vi "NicmosReverseScan.vi"(3 "Scan":T1, 7 "Reverse":bool, 9 "error out":errorcluster caption="error in (no error)") -> (0 "Reversed Scan":T1, 6 "error in (no error)":errorcluster caption="error out")   [LabVIEW 2009]
uses:
  Controls/NICMOS.DATA.ctl
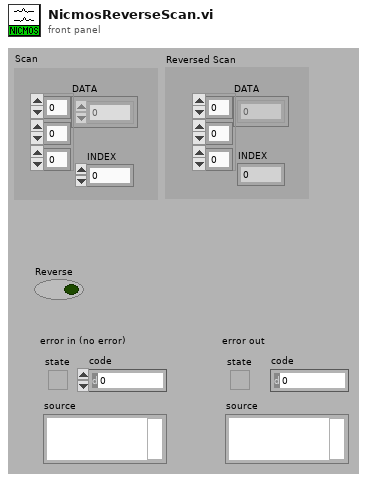
[diagram p1: front panel]
types:
  T1 = typedef "NICMOS.DATA.ctl" = cluster{"DATA":i32[][][], "INDEX":i32}
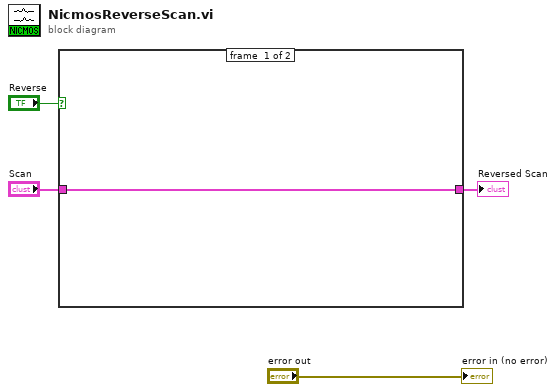
[diagram p0: block diagram]
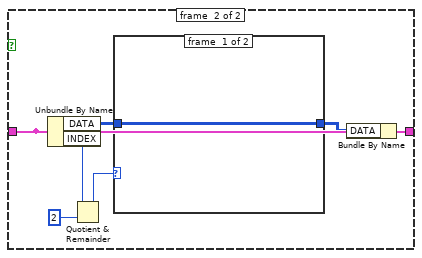
[diagram p2: hidden frame]
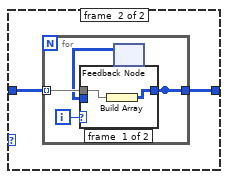
[diagram p3: hidden frame]
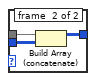
[diagram p4: hidden frame]
diagram:
  n1 = case shown="True" "Reverse" {
    tunnel: "Scan" -> [w5 w8]
    tunnel: [w5 w7] -> w3
    frame #0 {
    }
    frame #1 {
      n2 = Unbundle By Name(w8) -> ("DATA"=w9:i32[][][], "INDEX"=w10:i32)
      n3 = Quotient & Remainder(x=w10, y=2) -> (x-y*floor(x/y)=w12:i32)  [unwired: 1 out]
      n4 = case shown="1" w12 {
        tunnel: w9 -> [w13 w15]
        tunnel: [w13 w14] -> w6
        frame #0 {
        }
        frame #1 {
          n5 = for {
            tunnel: w15 -> [w17] mode=indexing
            tunnel: [w18] -> w14
            i -> [w19]
            n6 = feedback #1() -> (w16:i32[][][])  [unwired: 1 in]
            n7 = case shown="1, Default" w19 {
              tunnel: w16 -> [_ w24]
              tunnel: [w21 w23] -> w18
              tunnel: w17 -> [w20 w22]
              frame #0 {
                n8 = Build Array(w20) -> (w21:i32[][][])
              }
              frame #1 {
                n9 = Build Array (concatenate)(w22, w24) -> (w23:i32[][][])
              }
            }
          }
        }
      }
      n10 = Bundle By Name(cluster=w8, "DATA"=w6) -> (w7:T1)
    }
  }
  "Reversed Scan" <- w3
  "error in (no error)" <- "error out"
